vi "Check Delay Dependencies.vi"(6 "Problem Chnls in":string[](array[string]), 7 "BME_DG_System":refnum<class "BME_DG_System.lvclass">, 8 "error in (no error)":errorcluster, 9 "new Delay":dbl, 10 "Chnl":string, 11 "BME_DG_Chnl in":refnum<class "BME_DG_Chnl.lvclass">) -> (0 "error out":errorcluster, 2 "Dependecies OK":bool, 3 "BME_DG_Chnl out":refnum<class "BME_DG_Chnl.lvclass">, 4 "Problem Chnls out":string[](array[string]), 5 "BME_DG_System out":refnum<class "BME_DG_System.lvclass">)   [LabVIEW 2009, in "BME_DG_Chnl.lvclass"]
uses:
  BME_DG_Chnl.lvclass
  BME_DG_System/BME_DG_System.lvclass
  BME_DG_Chnl.lvclass/BME_DG_Chnl.ctl
  <vilib>/gmath/NI_Gmath.lvlib
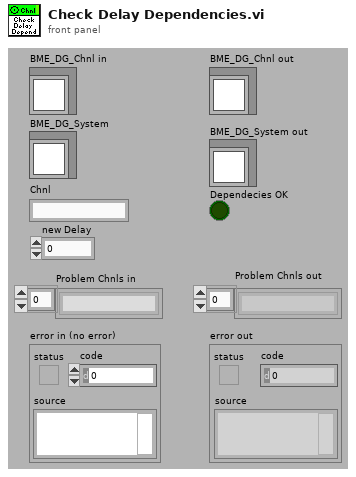
[diagram p1: front panel]
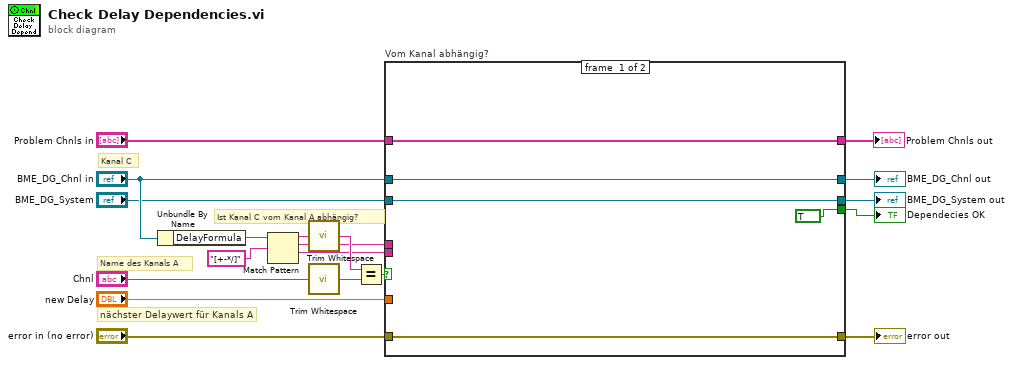
[diagram p0: block diagram]
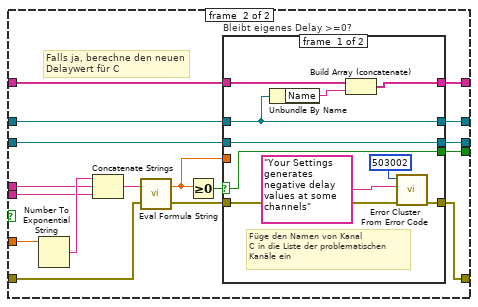
[diagram p2: hidden frame]
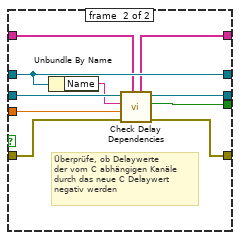
[diagram p3: hidden frame]
diagram:
  # "Ist Kanal C vom Kanal A abhängig?"
  # "nächster Delaywert für Kanals A"
  # "Name des Kanals A"
  # "Kanal C"
  n1 = Unbundle By Name("BME_DG_Chnl in") -> ("DelayFormula"=w13:string)
  n2 = Match Pattern(string=w13, regular expression="[+-*/]") -> (before substring=w15:string, match substring=w6:string, after substring=w5:string)  [unwired: 1 in, 1 out]
  n3 = call <vilib>:"Trim Whitespace.vi"("string"=w15) -> ("trimmed string"=w11:string)  [unwired: 1 in]
  n4 = call <vilib>:"Trim Whitespace.vi"("string"="Chnl") -> ("trimmed string"=w10:string)  [unwired: 1 in]
  n5 = Equal?(x=w11, y=w10) -> (x = y?=w9:bool)
  n6 = case "Vom Kanal abhängig?" shown="True" w9 {
    tunnel: "error in (no error)" -> [w21 w32]
    tunnel: [w21 w41] -> w18
    tunnel: [w24 w40] -> w17
    tunnel: "BME_DG_Chnl in" -> [w24 w39]
    tunnel: "BME_DG_System" -> [w23 w38]
    tunnel: "new Delay" -> [_ w36]
    tunnel: w6 -> [_ w34]
    tunnel: w5 -> [_ w33]
    tunnel: [TRUE ("Dependecies OK") w28] -> w3
    tunnel: [w23 w27] -> w4
    tunnel: "Problem Chnls in" -> [w20 w26]
    tunnel: [w20 w25] -> w1
    frame #0 {
    }
    frame #1 {
      # "Falls ja, berechne den neuen \nDelaywert für C"
      n7 = Number To Exponential String(number=w36) -> (E-format string=w35:string)  [unwired: 3 in]
      n8 = Concatenate Strings(w35, w34, w33) -> (w37:string)
      n9 = call <vilib>:"Eval Formula String.vi"("error in (no error)"=w32, "formula"=w37) -> ("error out"=w29:errorcluster, "y value"=w30:dbl)
      n10 = Greater Or Equal To 0?(x=w30) -> (x >= 0?=w31:bool)
      n11 = case "Bleibt eigenes Delay >=0?" shown="False" w31 {
        selector: w31 -> [w50 _]
        tunnel: [w44 w56] -> w41
        tunnel: [w47 w60] -> w40
        tunnel: w39 -> [w47 w60]
        tunnel: w38 -> [w49 w61]
        tunnel: w30 -> [_ w59]
        tunnel: w29 -> [w51 w58]
        tunnel: [w50 w55] -> w28
        tunnel: [w49 w57] -> w27
        tunnel: w26 -> [w48 w54]
        tunnel: [w45 w52] -> w25
        frame #0 {
          # "Füge den Namen von Kanal\nC in die Liste der problematischen\nKanäle ein"
          n12 = Unbundle By Name(w47) -> ("Name"=w46:string)
          n13 = Build Array (concatenate)(w48, w46) -> (w45:string[])
          n14 = call <vilib>:"Error Cluster From Error Code.vi"("error in (no error)"=w51, "error message (\"\")"="Your Settings generates negative delay values at some channels" ("error message (\"\")"), "error code (0)"=503002) -> ("error out"=w44:errorcluster)  [unwired: 6 in]
        }
        frame #1 {
          # "Überprüfe, ob Delaywerte\nder vom C abhängigen Kanäle\ndurch das neue C Delaywert \nnegativ werden"
          n15 = Unbundle By Name(w60) -> ("Name"=w53:string)
          n16 = call "Check Delay Dependencies.vi"("Problem Chnls in"=w54, "error in (no error)"=w58, "new Delay"=w59, "Chnl"=w53, "BME_DG_System in"=w61) -> ("error out"=w56:errorcluster, "Dependecies OK"=w55:bool, "BME_DG_System out"=w57:refnum<class "BME_DG_System.lvclass">, "Problem Chnls out"=w52:string[])  [unwired: 3 in]
        }
      }
    }
  }
  "error out" <- w18
  "BME_DG_Chnl out" <- w17
  "BME_DG_System out" <- w4
  "Dependecies OK" <- w3
  "Problem Chnls out" <- w1
